vi "read front panel string control.vi"(0 "VI Ref":refnum<vi>, 7 "control label":string, 11 "error in":errorcluster) -> (4 "dup VI Ref":refnum<vi>, 8 "string value":string, 15 "error out":errorcluster)   [LabVIEW 2020]
uses:
  <vilib>/Utility/traverseref.llb/TRef TravTarget.ctl
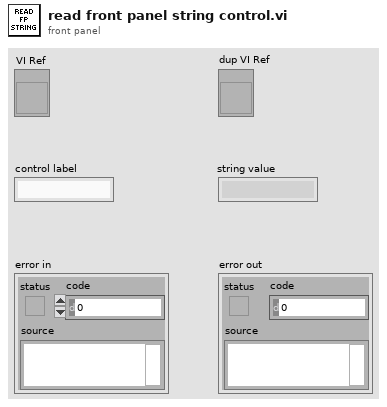
[diagram p1: front panel]
types:
  T1 = typedef "TRef TravTarget.ctl" = enum16{"FP", "BD", "Other"}
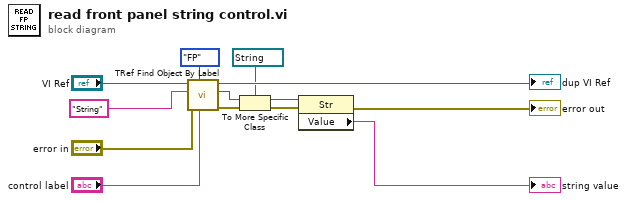
[diagram p0: block diagram]
diagram:
  n1 = call <vilib>:"TRef Find Object By Label.vi"("Label"="control label", "Traverse Target"=TRef_TravTarget."FP", "error in (no error)"="error in", "Class Name"="String", "VI Ref"="VI Ref") -> ("error out"=w10:errorcluster, "Found Obj Ref"=w8:refnum<vi>, "dup VI Ref"=→"dup VI Ref":refnum<vi>)  [unwired: 3 in, 1 out]
  n2 = To More Specific Class(target class=refnum<vi> refnum ("Other Refnum"), reference=w8, error in=w10) -> (specific class reference=w7:refnum<vi>, error out=w11:errorcluster)
  n3 = property class="Str"(reference=w7, error in=w11) -> (error out=→"error out":errorcluster, "Value"=→"string value":string)  [unwired: 1 out]
